vi "Read Double.vi"(8 "error in (no error)":errorcluster, 9 "Timeout (ms)":i32, 11 "CIFTag in":refnum<class "CIFTagDouble.lvclass">) -> (0 "error out":errorcluster, 1 "timed out?":bool, 2 "Data":dbl, 3 "CIFTag out":refnum<class "CIFTagDouble.lvclass">)   [LabVIEW 2021, in "CIFTagDouble.lvclass"]
uses:
  CIFTagDouble.lvclass
  D:/dev/CIF-LVCore/src/Channels/CIFChannels/CIFChannels.lvclass
  D:/dev/CIF-LVCore/src/Channels/CIFTag/CIFTag/CIFTag.lvclass
  CIFChannels/CIFChannels.lvclass/CIFChannels.ctl
  CIFChannels/Typedef/Channel State.ctl
  CIFChannels/Typedef/Direction.ctl
  CIFTagDouble.lvclass/CIFTagDouble.ctl
  CIFTag/CIFTag.lvclass/CIFTag.ctl
  cbead010-ab61-49ec-ac6c-083511305d37.vi
  CIFChannels/Accessors/Read Channel State.vi
  CIFChannels/Accessors/Read Direction.vi
  CIFChannels/Accessors/Write Channel State.vi
  CIFChannels/Accessors/Read Disconnect Behavior.vi
  cbead010-ab61-49ec-ac6c-083511305d37.vi/c28b0ead-42ad-4072-80a2-aca7f2bd7ce3.vi
  cbead010-ab61-49ec-ac6c-083511305d37.vi/219d0231-d98b-4193-b5cc-84f90e3c9091.vi
  <vilib>/CIFChannels/SubVIs/Get dll Path.vi
  CIFTag/CIFTag.lvclass
  CIFChannels/CIFChannels.lvclass
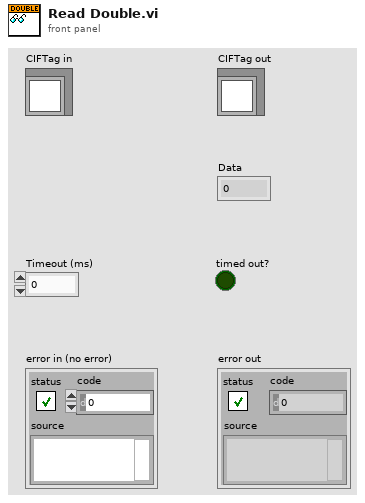
[diagram p1: front panel]
types:
  T1 = typedef "CIFChannels.lvclass/Channel State.ctl" = enum16{"Creating", "Disconnected", "Connecting", "Connected", "Destroyed"}
  T2 = typedef "CIFChannels.lvclass/Direction.ctl" = enum16{"Publisher", "Subscriber"}
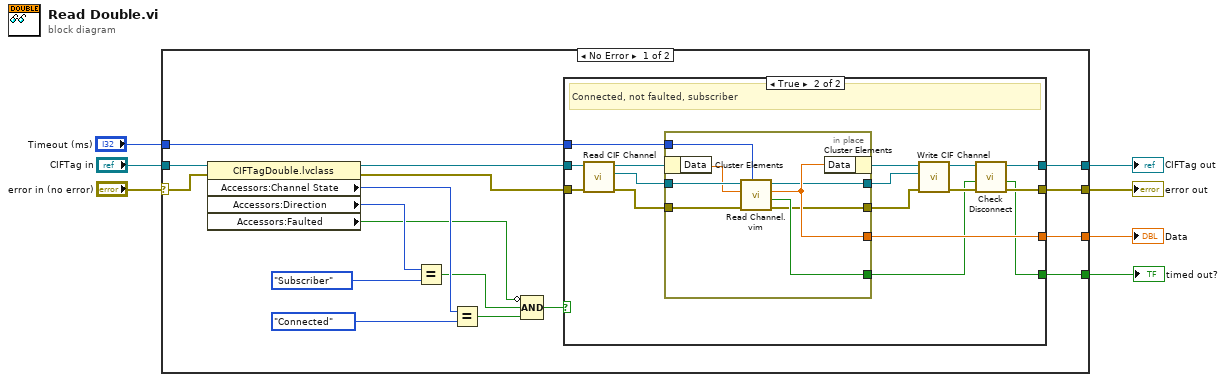
[diagram p0: block diagram]
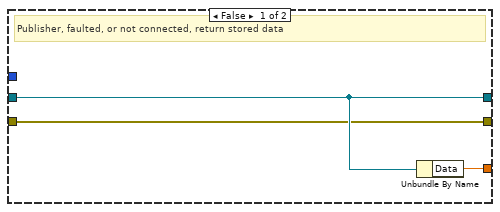
[diagram p2: hidden frame]
diagram:
  n1 = case shown="No Error" "error in (no error)" {
    selector: "error in (no error)" -> [w21 w53]
    tunnel: [w10 w53] -> w6
    tunnel: [w11 w52] -> w4
    tunnel: "CIFTag in" -> [w22 w52]
    tunnel: [w24 _] -> w3
    tunnel: [w23 _] -> w2
    tunnel: "Timeout (ms)" -> [w9 _]
    frame No Error {
      n2 = property class="CIFTagDouble.lvclass"(reference=w22, error in=w21) -> (reference out=w20:refnum<class "CIFTagDouble.lvclass">, error out=w19:errorcluster, "Accessors:Channel State"=w16:T1, "Accessors:Direction"=w18:T2, "Accessors:Faulted"=w8:bool)
      n3 = Equal?(x=w18, y=Direction."Subscriber") -> (x = y?=w12:bool)
      n4 = Equal?(x=w16, y=Channel_State."Connected") -> (x = y?=w14:bool)
      n5 = Compound Arithmetic op=AND(invert w8, w12, w14) -> (w13:bool)
      n6 = case shown="True" w13 {
        tunnel: [_ w29] -> w24
        tunnel: [w27 w36] -> w23
        tunnel: w19 -> [w25 w42]
        tunnel: w20 -> [w26 w43]
        tunnel: [w26 w41] -> w11
        tunnel: [w25 w40] -> w10
        tunnel: w9 -> [_ w28]
        frame False {
          # "Publisher, faulted, or not connected, return stored data"
          n7 = Unbundle By Name(w26) -> ("Data"=w27:dbl)
        }
        frame True {
          # "Connected, not faulted, subscriber"
          n8 = call "Read CIF Channel.vi"("error in (no error)"=w42, "CIFTag in"=w43) -> ("error out"=w37:errorcluster, "CIF Channel"=w38:refnum<k21>, "CIFTag out"=w39:refnum<class "CIFTagDouble.lvclass">)  [unwired: 7 in]
          n9 = in-place {
            in-place-border: [w48] -> w30
            in-place-border: w38 -> [w51]
            in-place-border: w37 -> [w49]
            in-place-border: [w47] -> w36
            in-place-border: [w46] -> w33
            in-place-border: [w45] -> w34
            in-place-border: w28 -> [w44]
            n10 = in-place-cluster #1(w39) -> ("Data"=w50:dbl)
            n11 = call "Read Channel.vim"("Timeout (ms)"=w44, "error in"=w49, "Data in"=w50, "CIF Channel in"=w51) -> ("error out"=w45:errorcluster, "Timed out?"=w48:bool, "Data out"=w47:dbl, "CIF Channel out"=w46:refnum<k21>)  [unwired: 4 in]
            n12 = in-place-cluster #1("Data"=w47) -> (w35:refnum<class "CIFTagDouble.lvclass">)
          }
          n13 = call "Write CIF Channel.vi"("error in (no error)"=w34, "CIF Channel"=w33, "CIFTag in"=w35) -> ("error out"=w31:errorcluster, "CIFTag out"=w32:refnum<class "CIFTagDouble.lvclass">)  [unwired: 7 in]
          n14 = call "Check Disconnect.vi"("error in (no error)"=w31, "timeout in"=w30, "CIFTag in"=w32) -> ("error out"=w40:errorcluster, "timeout out"=w29:bool, "CIFTag out"=w41:refnum<class "CIFTagDouble.lvclass">)  [unwired: 5 in, 1 out]
        }
      }
    }
    frame Error {
    }
  }
  "error out" <- w6
  "CIFTag out" <- w4
  "timed out?" <- w3
  "Data" <- w2
